vi "execute.vi"(8 "error in (no error)":errorcluster, 11 "UpdateDL090216DisplayCommand in":refnum<class "UpdateDisplayDL090216Command.lvclass">) -> (0 "error out":errorcluster, 3 "UpdateDL090216DisplayCommand out":refnum<class "UpdateDisplayDL090216Command.lvclass">)   [LabVIEW 2010, in "UpdateDisplayDL090216Command.lvclass"]
uses:
  UpdateDisplayDL090216Command.lvclass
  DisplayDL090216/DisplayDL090216.lvclass
  GenericDisplay/GenericDisplay/GenericDisplay.lvclass
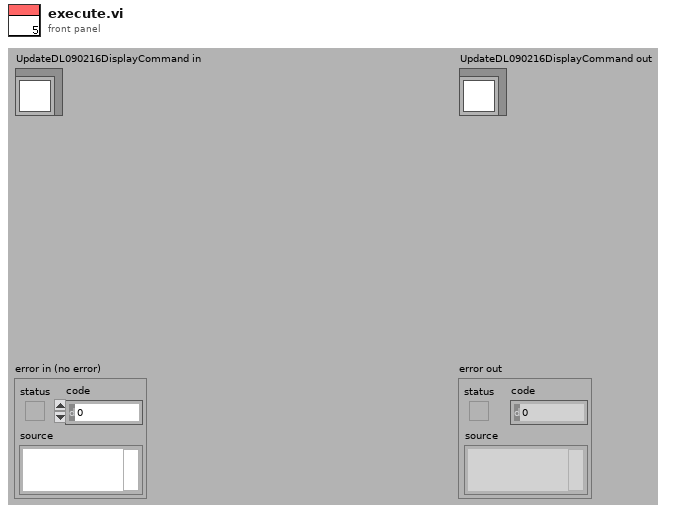
[diagram p1: front panel]
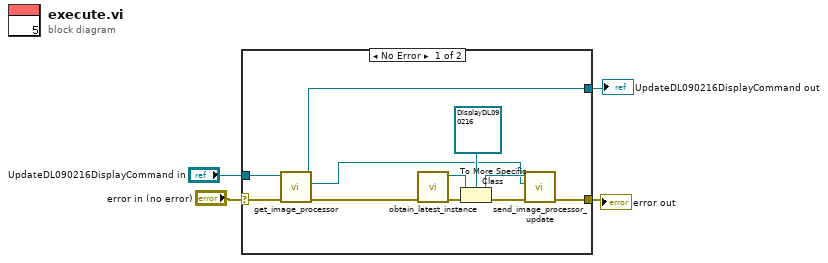
[diagram p0: block diagram]
diagram:
  n1 = case shown="No Error" "error in (no error)" {
    selector: "error in (no error)" -> [w9 w17]
    tunnel: [w15 w17] -> w3
    tunnel: [w10 w16] -> w1
    tunnel: "UpdateDL090216DisplayCommand in" -> [w11 w16]
    frame No Error {
      n2 = call-dynamic "get_image_processor.vi"("error in (no error)"=w9, "GenericImageProcessorChangedCommand.lvclass in"=w11) -> ("error out"=w5:errorcluster, "image processor"=w8:refnum<class "GenericImageProcessor.lvclass">, "GenericImageProcessorChangedCommand.lvclass out"=w10:refnum<class "UpdateDisplayDL090216Command.lvclass">)  [unwired: 7 out]
      n3 = call "obtain_latest_instance.vi"("error in (no error)"=w5) -> ("error out"=w7:errorcluster, "GenericDisplay out"=w6:refnum<class "GenericDisplay.lvclass">)  [unwired: 1 in, 8 out]
      n4 = To More Specific Class(target class=refnum<class "DisplayDL090216.lvclass"> refnum ("DL090216Display.lvclass"), reference=w6, error in=w7) -> (specific class reference=w13:refnum<class "DisplayDL090216.lvclass">, error out=w12:errorcluster)
      n5 = call-dynamic "send_image_processor_update.vi"("error in (no error)"=w12, "image processor update"=w8, "DL090216Display in"=w13) -> ("error out"=w15:errorcluster)  [unwired: 8 out]
    }
    frame Error {
    }
  }
  "error out" <- w3
  "UpdateDL090216DisplayCommand out" <- w1
